vi "Double FFT Mesurament RT with Frequency Linearization.vi"() -> ()   [LabVIEW 2014]
uses:
  <vilib>/Platform/TimedLoop/XDataNode/timing_clust.ctl
  <vilib>/Platform/TimedLoop/XDataNode/nitl_modes.ctl
  <vilib>/Platform/TimedLoop/XDataNode/wakeup.ctl
  <vilib>/FPGAPlugInAG/sbRIO-9636/niLvFpga_Open_sbRIO-9636.vi
  <vilib>/rvi/interface/common/dynamic/niFpgaDynamicAddResources.vi
  <vilib>/Utility/error.llb/Error Cluster From Error Code.vi
  <vilib>/rvi/errors/niLvFpgaAdjustHostInterfaceError.vi
  <vilib>/rvi/interface/common/niFpgaWaitOnOcc.vi
  <vilib>/FPGAPlugInAG/Dynamic/niLvFpga_Run_Dynamic.vi
  <vilib>/FPGAPlugInAG/Dynamic/niLvFpga_Abort_Dynamic.vi
  <vilib>/FPGAPlugInAG/Dynamic/niLvFpga_Reset_Dynamic.vi
  <vilib>/FPGAPlugInAG/Dynamic/niLvFpga_Close_Dynamic.vi
  <vilib>/rvi/interface/nirviOpenFPGA/nirviOpenFPGA.xnode
  FPGA Bitfiles/LaserDistanceSen_FPGATarget_DoubleFFTMesuram_r82pz3ZO4sk.lvbitx
  FPGA Target/Test VIs/Double FFT Mesurament Test.vi
  FPGA Bitfiles/LaserDistanceSen_FPGATarget_DoubleFFTMesuram_atjrRfXVdPQ.lvbitx
  FPGA Target/Test VIs/Double FFT Mesurament Test SLOW.vi
  <vilib>/rvi/interface/nirviReadWriteControl/nirviReadWriteControl.xnode
  <vilib>/rvi/interface/nirviMethod/nirviMethod.xnode
  <vilib>/Platform/TimedLoop/XDataNode/XDataNode.xnode
  <vilib>/rvi/interface/nirviCloseFPGA/nirviCloseFPGA.xnode
  <vilib>/FPGAPlugInAG/Dynamic/niLvFpga_ConfigureFifo_Dynamic.vi
  <vilib>/rvi/errors/niLvFpgaMergeErrorWithErrorCode.vi
  <vilib>/FPGAPlugInAG/Dynamic/niLvFpga_StartFifo_Dynamic.vi
  <vilib>/rvi/interface/Simulation/niFpgaSimulationCallBeginRW.vi
  <vilib>/FPGAPlugInAG/Dynamic/niLvFpga_ReadFifo_Dynamic.vi
  <vilib>/Platform/TimedLoop/XDataNode/XDNodeRunTimeDep.lvlib
  NiFpgaLv.dll
panel:
  in  "Active PolyFit":bool
  out "2) Max-Min error":dbl
  out "1) Max-Min error":dbl
  in  "Sample /Modulation Frequency":enum32{"40MHz/32KHz", "30MHz/24Khz"}(radio)=enum."30MHz/24Khz"
  in  "Scaling Factor":dbl=1.0
  in  "Scale Factor Rising":dbl=0.5
  out "2) Std Dev":dbl
  out "1) Std Dev":dbl
  in  "Scale Factor Falling":dbl=0.5
  in  "Triangolo dritto":bool=TRUE
  in  "Acrive  Smooth":bool
  out "Complete SkewTri":dbl[](graph)
  out "2) Tri edge RISING":dbl[](graph)
  out "1) Tri edge FALLING":dbl[](graph)
  out "1) Ext Mean Time Curve":dbl[](graph)
  out "2) Ext Mean Time Curve":dbl[](graph)
  out "2) Mean Freq Curve Rising":dbl[](graph)
  out "1) Mean Freq Curve Falling":dbl[](graph)
  out "2) Freq curve":dbl[](graph)
  out "1) Freq curve":dbl[](graph)
  in  "FFT Sliding Win Size":i32=128
  out "1) SmoothSubSig":dbl[](graph)
  out "2) SmoothSubSig":dbl[](graph)
  in  "Acrive Fit":bool=TRUE
  in  "Poly Order":i32=3
  in  "Side points":i32=13
  in  "Poly Grade":dbl=5.0
  out "2) Signal&Fit 2":dbl[][](graph)
  out "1) Signal&Fit":dbl[][](graph)
  in  "tieni premuto per":i32=1
  out "Current Sig lin":i32
  in  "Acrive Linearization":bool
  in  "# Measurements for Linearization":i32=10
  in  "?":bool
  out "maxbin_secondFFT":i32
  out "maxbin_firstFFT":i32
  out "f_rise":dbl
  out "f_fall":dbl
  out "f_mean":dbl
  out "Velocity (m/s)":dbl
  out "Distance (m)":dbl
  in  "Initial Latency points":u32(slide) scale=0.0..1249.0
  out "Second FFT (bin)":dbl[](graph)
  out "Second Signal (points) - Rising Triangular":dbl[](graph)
  out "First FFT (bin)":dbl[](graph)
  out "First Signal (points) - Falling Triangular":dbl[](graph)
  in  "Snapshot":bool
  in  "Windowing":T1(ring)
  in  "first bin":i32=5
  in  "last bin":i32=255
  in  "lower limit 2":u32(slide)=738 scale=625.0..738.0
  in  "lower limit 1":u32(slide)=113 scale=0.0..113.0
  # "OFFLINE parameters"
  # "WARNING:\nOnce pressed wait untill the end of operation"
  # "Triangolo storto\nda costante"
  # "Max Detection FFT bin range"
  # "ONLINE parameters"
  # "Se la sottrazione del fondo non è eseguita su FPGA.\n Attivarla per eseguirla lato RT"
  # "Smoothing (S-G Params)"
  # "Fitting"
  # "ONLY POWER OF 2"
  # "Min: 2 Max: 256 (2, 4, 8, 16, 32, 64, 128, 256)"
  # "LINEARIZATION FINAL RESULTS"
  # "%"
  # "%"
  # "% over Mean"
  # "% over Mean"
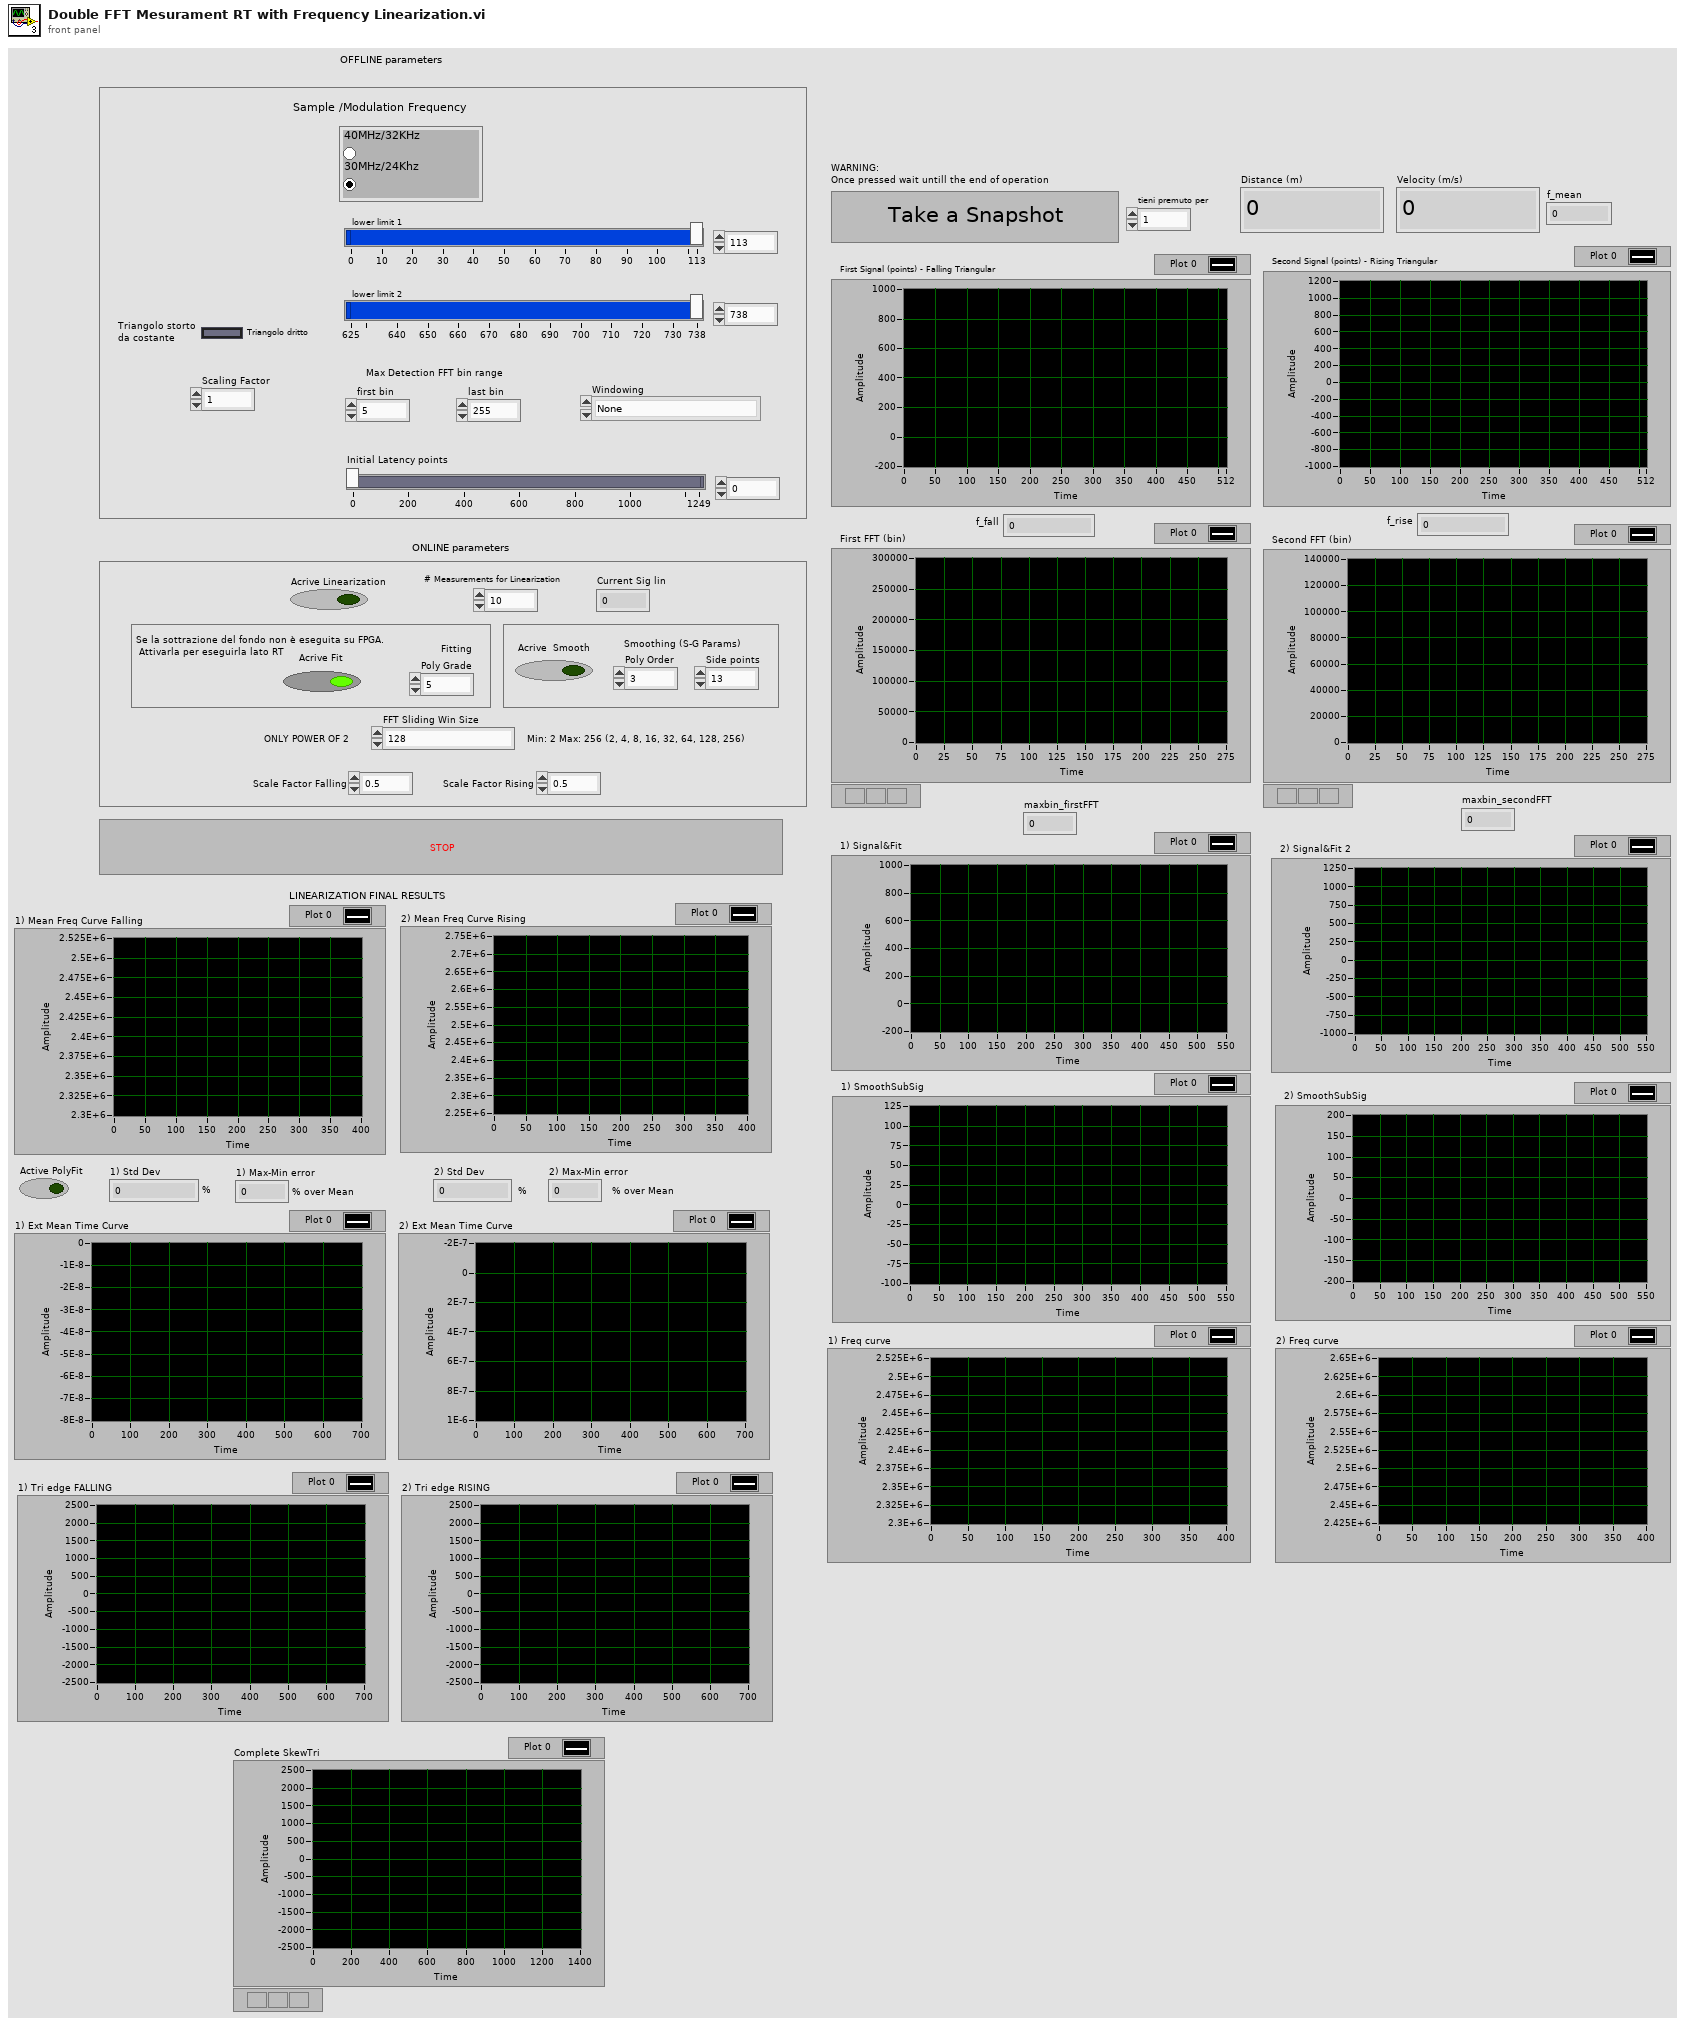
[diagram p1: front panel]
types:
  T1 = enum16{"None", "Hanning", "Hamming", "Blackman", "Blackman-Harris"}
  T2 = typedef "XDNodeRunTimeDep.lvlib/timing_clust.ctl" = cluster{"Expected End [f-1]":u64, "Actual End [f-1]":u64, "Finished Late? [f-1]":bool, "Expected End [i-1]":u64, "Actual End [i-1]":u64, "Finished Late? [i-1]":bool, "Expected Start [i]":u64, "Actual Start [i]":u64, "Expected Start [f]":u64, "Actual Start [f]":u64, "Source Name":string, "Structure Name":string, "Period":i64, "Deadline":i64, "Offset":i64, "Start":i64, "Priority":i32, "Timeout":i32, "Mode":T3, "Wakeup Reason":T4, "Error":errorcluster, "Source Type":string, "Secondary Source Type":string, "Global End Time":u64, "Global Start Time":u64, "Frame Duration":u64, "Iteration Duration":u64, "Assigned CPU":i32, "I/O Scan Engine Mode":u32}
  T3 = typedef "XDNodeRunTimeDep.lvlib/nitl_modes.ctl" = enum32{"No Change", "Process missed periods, maintain original phase", "Discard missed periods, maintain original phase", "Process missed periods, ignore original phase", "Discard missed periods, ignore original phase"}
  T4 = typedef "XDNodeRunTimeDep.lvlib/wakeup.ctl" = enum32{"Normal", "Aborted", "Asynchronous wakeup", "Timing source error", "Timed loop error", "Timeout"}
  T5 = typedef "NI_Matrix.lvlib/RealMatrix.ctl" = dbl[][]
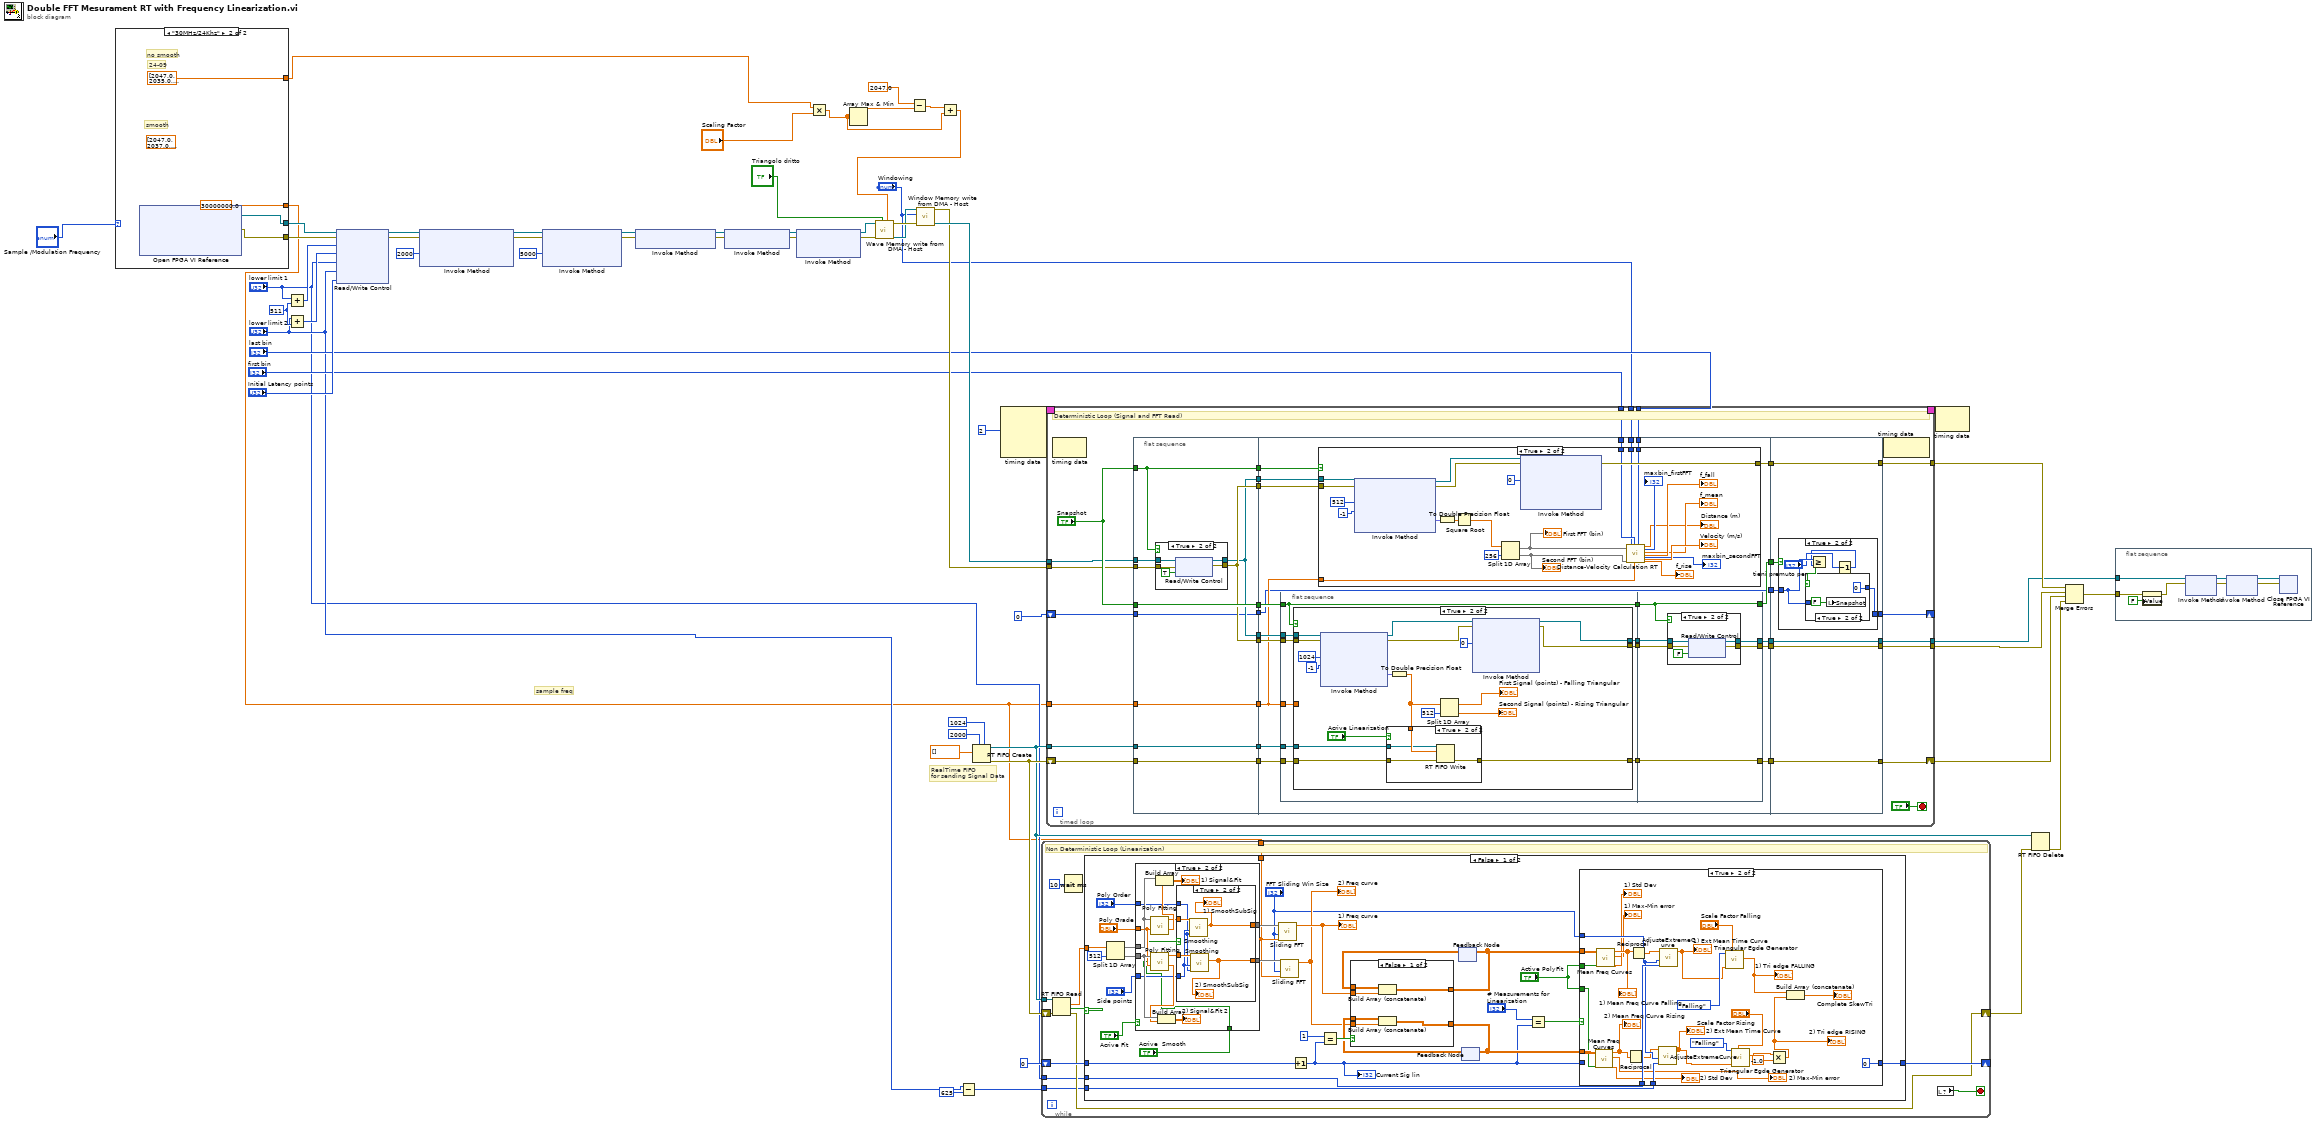
[diagram p0: block diagram]
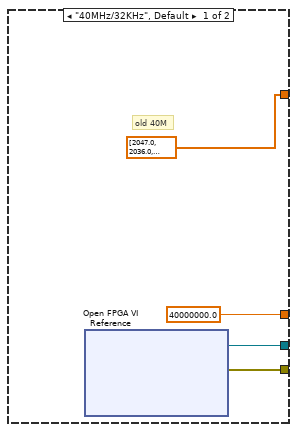
[diagram p2: hidden frame]
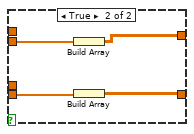
[diagram p6: hidden frame]
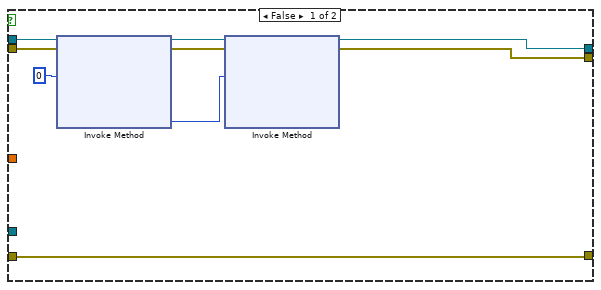
[diagram p9: hidden frame]
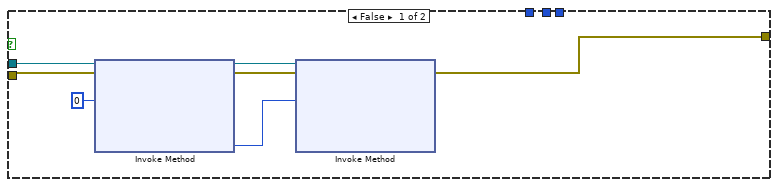
[diagram p12: hidden frame]
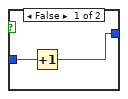
[diagram p14: hidden frame]
diagram:
  w56 = u32 511 ("y")
  # "sample freq"
  # "RealTime FIFO \nfor sending Signal Data"
  n1 = case shown="\"30MHz/24Khz\"" "Sample /Modulation Frequency" {
    tunnel: [w62 w65] -> w55
    tunnel: [w61 w66] -> w54
    tunnel: [40000000.0 30000000.0] -> w2
    tunnel: [dbl[] [2047.0, 2036.0, 2024.0, 2013.0, 2002.0, 1990.0, 1979.0, 1968.0, 1956.0, 1945.0, 1934.0, 1923.0, 1912.0, 1900.0, 1889.0, 1878.0, 1867.0, 1856.0, 1845.0, 1833.0, 1822.0, 1811.0, 1800.0, 1789.0, 1778.0, 1767.0, 1756.0, 1745.0, 1734.0, 1723.0, 1712.0, 1702.0, 1691.0, 1680.0, 1669.0, 1658.0, 1647.0, 1636.0, 1626.0, 1615.0, 1604.0, 1593.0, 1583.0, 1572.0, 1561.0, 1550.0, 1540.0, 1529.0, 1518.0, 1508.0, 1497.0, 1487.0, 1476.0, 1465.0, 1455.0, 1444.0, 1434.0, 1423.0, 1413.0, 1402.0, 1392.0, 1381.0, 1371.0, 1360.0, 1350.0, 1340.0, 1329.0, 1319.0, 1309.0, 1298.0, 1288.0, 1278.0, 1267.0, 1257.0, 1247.0, 1237.0, 1226.0, 1216.0, 1206.0, 1196.0, 1186.0, 1176.0, 1165.0, 1155.0, 1145.0, 1135.0, 1125.0, 1115.0, 1105.0, 1095.0, 1085.0, 1075.0, 1065.0, 1055.0, 1045.0, 1035.0, 1025.0, 1015.0, 1006.0, 996.0, 986.0, 976.0, 966.0, 956.0, 947.0, 937.0, 927.0, 917.0, 908.0, 898.0, 888.0, 879.0, 869.0, 859.0, 850.0, 837.0, 826.0, 816.0, 804.0, 796.0, 788.0, 778.0, 769.0, 758.0, 750.0, 743.0, 733.0, 724.0, 717.0, 709.0, 701.0, 693.0, 686.0, 677.0, 669.0, 661.0, 653.0, 645.0, 638.0, 630.0, 622.0, 615.0, 607.0, 599.0, 592.0, 583.0, 576.0, 569.0, 561.0, 554.0, 547.0, 539.0, 532.0, 525.0, 518.0, 509.0, 501.0, 492.0, 486.0, 478.0, 471.0, 463.0, 456.0, 450.0, 442.0, 435.0, 429.0, 421.0, 415.0, 408.0, 401.0, 394.0, 388.0, 381.0, 375.0, 368.0, 361.0, 355.0, 349.0, 342.0, 336.0, 330.0, 323.0, 317.0, 311.0, 304.0, 298.0, 292.0, 286.0, 279.0, 273.0, 267.0, 261.0, 255.0, 249.0, 242.0, 236.0, 230.0, 224.0, 218.0, 212.0, 206.0, 200.0, 194.0, 187.0, 181.0, 175.0, 169.0, 163.0, 157.0, 150.0, 144.0, 138.0, 132.0, 125.0, 119.0, 113.0, 107.0, 101.0, 95.0, 88.0, 82.0, 77.0, 71.0, 65.0, 59.0, 53.0, 47.0, 41.0, 35.0, 29.0, 23.0, 18.0, 11.0, 6.0, 0.0, -6.0, -12.0, -18.0, -23.0, -29.0, -35.0, -41.0, -47.0, -52.0, -58.0, -64.0, -69.0, -75.0, -81.0, -87.0, -92.0, -98.0, -104.0, -109.0, -115.0, -121.0, -126.0, -132.0, -138.0, -144.0, -149.0, -155.0, -161.0, -166.0, -172.0, -177.0, -183.0, -189.0, -194.0, -200.0, -205.0, -211.0, -216.0, -222.0, -227.0, -233.0, -238.0, -244.0, -249.0, -255.0, -260.0, -266.0, -271.0, -277.0, -283.0, -288.0, -294.0, -299.0, -304.0, -310.0, -315.0, -321.0, -326.0, -331.0, -337.0, -342.0, -348.0, -353.0, -358.0, -364.0, -369.0, -375.0, -380.0, -385.0, -391.0, -396.0, -402.0, -407.0, -413.0, -418.0, -423.0, -429.0, -434.0, -439.0, -445.0, -450.0, -456.0, -461.0, -466.0, -472.0, -477.0, -483.0, -488.0, -493.0, -499.0, -504.0, -510.0, -515.0, -520.0, -526.0, -531.0, -537.0, -542.0, -548.0, -553.0, -558.0, -564.0, -569.0, -574.0, -580.0, -585.0, -590.0, -596.0, -601.0, -606.0, -612.0, -617.0, -622.0, -628.0, -633.0, -638.0, -644.0, -649.0, -654.0, -660.0, -665.0, -670.0, -676.0, -681.0, -686.0, -692.0, -697.0, -702.0, -708.0, -713.0, -718.0, -723.0, -729.0, -734.0, -739.0, -744.0, -750.0, -755.0, -760.0, -765.0, -771.0, -776.0, -781.0, -786.0, -792.0, -797.0, -802.0, -807.0, -812.0, -818.0, -823.0, -828.0, -833.0, -839.0, -844.0, -849.0, -854.0, -859.0, -865.0, -870.0, -875.0, -880.0, -885.0, -891.0, -896.0, -901.0, -906.0, -911.0, -916.0, -922.0, -927.0, -932.0, -937.0, -943.0, -948.0, -953.0, -958.0, -963.0, -969.0, -974.0, -979.0, -984.0, -989.0, -995.0, -1000.0, -1005.0, -1010.0, -1015.0, -1021.0, -1026.0, -1031.0, -1036.0, -1041.0, -1047.0, -1052.0, -1057.0, -1062.0, -1067.0, -1073.0, -1078.0, -1083.0, -1088.0, -1093.0, -1099.0, -1104.0, -1109.0, -1114.0, -1119.0, -1124.0, -1130.0, -1135.0, -1140.0, -1145.0, -1150.0, -1156.0, -1161.0, -1166.0, -1171.0, -1176.0, -1182.0, -1187.0, -1192.0, -1197.0, -1202.0, -1207.0, -1213.0, -1218.0, -1223.0, -1228.0, -1233.0, -1238.0, -1244.0, -1249.0, -1254.0, -1259.0, -1264.0, -1269.0, -1275.0, -1280.0, -1285.0, -1290.0, -1295.0, -1300.0, -1305.0, -1311.0, -1316.0, -1321.0, -1326.0, -1331.0, -1336.0, -1342.0, -1347.0, -1352.0, -1357.0, -1362.0, -1367.0, -1372.0, -1378.0, -1383.0, -1388.0, -1393.0, -1398.0, -1403.0, -1408.0, -1414.0, -1419.0, -1424.0, -1429.0, -1434.0, -1439.0, -1444.0, -1450.0, -1455.0, -1460.0, -1465.0, -1470.0, -1475.0, -1480.0, -1486.0, -1491.0, -1496.0, -1501.0, -1506.0, -1511.0, -1516.0, -1522.0, -1527.0, -1532.0, -1537.0, -1542.0, -1547.0, -1552.0, -1558.0, -1563.0, -1568.0, -1573.0, -1578.0, -1583.0, -1588.0, -1593.0, -1599.0, -1604.0, -1609.0, -1614.0, -1619.0, -1624.0, -1629.0, -1634.0, -1640.0, -1645.0, -1650.0, -1655.0, -1660.0, -1665.0, -1670.0, -1675.0, -1681.0, -1686.0, -1691.0, -1696.0, -1701.0, -1706.0, -1711.0, -1716.0, -1722.0, -1727.0, -1732.0, -1737.0, -1742.0, -1747.0, -1752.0, -1757.0, -1762.0, -1768.0, -1773.0, -1778.0, -1783.0, -1788.0, -1793.0, -1798.0, -1803.0, -1808.0, -1814.0, -1819.0, -1824.0, -1829.0, -1834.0, -1839.0, -1844.0, -1849.0, -1854.0, -1859.0, -1865.0, -1870.0, -1875.0, -1880.0, -1885.0, -1890.0, -1895.0, -1900.0, -1905.0, -1911.0, -1916.0, -1921.0, -1926.0, -1931.0, -1936.0, -1941.0, -1946.0, -1951.0, -1956.0, -1961.0, -1967.0, -1972.0, -1977.0, -1982.0, -1987.0, -1992.0, -1997.0, -2002.0, -2007.0, -2012.0, -2017.0, -2023.0, -2028.0, -2033.0, -2038.0, -2043.0, -2048.0, -2047.0, -2034.0, -2021.0, -2009.0, -1996.0, -1983.0, -1970.0, -1957.0, -1945.0, -1932.0, -1919.0, -1907.0, -1894.0, -1881.0, -1869.0, -1856.0, -1844.0, -1831.0, -1819.0, -1806.0, -1794.0, -1781.0, -1769.0, -1757.0, -1744.0, -1732.0, -1719.0, -1707.0, -1695.0, -1682.0, -1670.0, -1658.0, -1646.0, -1634.0, -1621.0, -1609.0, -1597.0, -1585.0, -1573.0, -1561.0, -1549.0, -1537.0, -1525.0, -1513.0, -1501.0, -1489.0, -1477.0, -1465.0, -1453.0, -1441.0, -1429.0, -1417.0, -1405.0, -1394.0, -1382.0, -1370.0, -1358.0, -1347.0, -1335.0, -1323.0, -1312.0, -1300.0, -1288.0, -1277.0, -1265.0, -1254.0, -1242.0, -1231.0, -1219.0, -1208.0, -1196.0, -1185.0, -1173.0, -1162.0, -1150.0, -1139.0, -1128.0, -1116.0, -1105.0, -1094.0, -1083.0, -1071.0, -1060.0, -1049.0, -1038.0, -1027.0, -1015.0, -1004.0, -993.0, -982.0, -971.0, -960.0, -949.0, -938.0, -927.0, -916.0, -905.0, -894.0, -883.0, -873.0, -862.0, -851.0, -840.0, -829.0, -819.0, -808.0, -797.0, -786.0, -776.0, -765.0, -754.0, -744.0, -733.0, -722.0, -712.0, -697.0, -685.0, -674.0, -661.0, -652.0, -643.0, -632.0, -622.0, -610.0, -602.0, -594.0, -583.0, -574.0, -566.0, -558.0, -550.0, -542.0, -534.0, -525.0, -516.0, -507.0, -499.0, -491.0, -483.0, -475.0, -467.0, -459.0, -451.0, -443.0, -435.0, -426.0, -419.0, -411.0, -404.0, -396.0, -388.0, -381.0, -373.0, -366.0, -359.0, -349.0, -341.0, -331.0, -325.0, -317.0, -309.0, -301.0, -295.0, -288.0, -280.0, -273.0, -266.0, -259.0, -252.0, -246.0, -239.0, -231.0, -225.0, -219.0, -212.0, -205.0, -199.0, -192.0, -186.0, -180.0, -173.0, -167.0, -161.0, -155.0, -148.0, -142.0, -136.0, -130.0, -124.0, -118.0, -112.0, -106.0, -100.0, -94.0, -88.0, -82.0, -76.0, -70.0, -64.0, -58.0, -52.0, -46.0, -40.0, -34.0, -28.0, -21.0, -15.0, -9.0, -3.0, 2.0, 9.0, 15.0, 21.0, 27.0, 33.0, 39.0, 45.0, 51.0, 57.0, 63.0, 69.0, 75.0, 81.0, 86.0, 92.0, 98.0, 103.0, 110.0, 116.0, 121.0, 127.0, 133.0, 138.0, 144.0, 149.0, 155.0, 161.0, 166.0, 172.0, 177.0, 183.0, 189.0, 194.0, 200.0, 205.0, 211.0, 216.0, 221.0, 227.0, 232.0, 238.0, 243.0, 249.0, 254.0, 259.0, 265.0, 270.0, 276.0, 281.0, 286.0, 292.0, 297.0, 303.0, 308.0, 314.0, 319.0, 324.0, 329.0, 335.0, 340.0, 345.0, 351.0, 356.0, 361.0, 366.0, 371.0, 377.0, 382.0, 387.0, 392.0, 397.0, 403.0, 408.0, 413.0, 418.0, 423.0, 429.0, 434.0, 439.0, 444.0, 449.0, 454.0, 459.0, 464.0, 469.0, 474.0, 479.0, 484.0, 489.0, 494.0, 499.0, 504.0, 509.0, 514.0, 520.0, 525.0, 530.0, 535.0, 540.0, 545.0, 550.0, 555.0, 560.0, 565.0, 570.0, 575.0, 580.0, 585.0, 590.0, 595.0, 600.0, 605.0, 610.0, 615.0, 620.0, 625.0, 630.0, 636.0, 641.0, 646.0, 651.0, 656.0, 661.0, 666.0, 671.0, 676.0, 681.0, 686.0, 691.0, 696.0, 701.0, 706.0, 711.0, 716.0, 721.0, 726.0, 731.0, 736.0, 741.0, 746.0, 751.0, 756.0, 761.0, 765.0, 770.0, 775.0, 780.0, 785.0, 790.0, 795.0, 800.0, 805.0, 810.0, 815.0, 820.0, 825.0, 829.0, 834.0, 839.0, 844.0, 849.0, 854.0, 859.0, 864.0, 868.0, 873.0, 878.0, 883.0, 888.0, 893.0, 897.0, 902.0, 907.0, 912.0, 917.0, 921.0, 926.0, 931.0, 936.0, 941.0, 945.0, 950.0, 955.0, 960.0, 965.0, 969.0, 974.0, 979.0, 984.0, 988.0, 993.0, 998.0, 1003.0, 1007.0, 1012.0, 1017.0, 1022.0, 1027.0, 1031.0, 1036.0, 1041.0, 1046.0, 1051.0, 1055.0, 1060.0, 1065.0, 1070.0, 1075.0, 1079.0, 1084.0, 1089.0, 1094.0, 1098.0, 1103.0, 1108.0, 1113.0, 1118.0, 1122.0, 1127.0, 1132.0, 1137.0, 1141.0, 1146.0, 1151.0, 1156.0, 1161.0, 1165.0, 1170.0, 1175.0, 1180.0, 1184.0, 1189.0, 1194.0, 1199.0, 1204.0, 1208.0, 1213.0, 1218.0, 1223.0, 1227.0, 1232.0, 1237.0, 1242.0, 1246.0, 1251.0, 1256.0, 1261.0, 1265.0, 1270.0, 1275.0, 1280.0, 1284.0, 1289.0, 1294.0, 1299.0, 1303.0, 1308.0, 1313.0, 1318.0, 1322.0, 1327.0, 1332.0, 1336.0, 1341.0, 1346.0, 1351.0, 1355.0, 1360.0, 1365.0, 1370.0, 1374.0, 1379.0, 1384.0, 1388.0, 1393.0, 1398.0, 1403.0, 1407.0, 1412.0, 1417.0, 1421.0, 1426.0, 1431.0, 1436.0, 1440.0, 1445.0, 1450.0, 1454.0, 1459.0, 1464.0, 1469.0, 1473.0, 1478.0, 1483.0, 1487.0, 1492.0, 1497.0, 1502.0, 1506.0, 1511.0, 1516.0, 1520.0, 1525.0, 1530.0, 1535.0, 1539.0, 1544.0, 1549.0, 1553.0, 1558.0, 1563.0, 1567.0, 1572.0, 1577.0, 1582.0, 1586.0, 1591.0, 1596.0, 1600.0, 1605.0, 1610.0, 1614.0, 1619.0, 1624.0, 1628.0, 1633.0, 1638.0, 1643.0, 1647.0, 1652.0, 1657.0, 1661.0, 1666.0, 1671.0, 1675.0, 1680.0, 1685.0, 1689.0, 1694.0, 1699.0, 1703.0, 1708.0, 1713.0, 1717.0, 1722.0, 1727.0, 1731.0, 1736.0, 1741.0, 1746.0, 1750.0, 1755.0, 1760.0, 1764.0, 1769.0, 1774.0, 1778.0, 1783.0, 1788.0, 1792.0, 1797.0, 1802.0, 1806.0, 1811.0, 1816.0, 1820.0, 1825.0, 1830.0, 1834.0, 1839.0, 1844.0, 1848.0, 1853.0, 1858.0, 1862.0, 1867.0, 1871.0, 1876.0, 1881.0, 1885.0, 1890.0, 1895.0, 1899.0, 1904.0, 1909.0, 1913.0, 1918.0, 1923.0, 1927.0, 1932.0, 1937.0, 1941.0, 1946.0, 1951.0, 1955.0, 1960.0, 1965.0, 1969.0, 1974.0, 1978.0, 1983.0, 1988.0, 1992.0, 1997.0, 2002.0, 2006.0, 2011.0, 2016.0, 2020.0, 2025.0, 2029.0, 2034.0, 2039.0, 2043.0, 2048.0] ("Complete SkewTri") dbl[] [2047.0, 2035.0, 2022.0, 2010.0, 1997.0, 1985.0, 1972.0, 1960.0, 1948.0, 1935.0, 1923.0, 1911.0, 1899.0, 1886.0, 1874.0, 1862.0, 1850.0, 1838.0, 1825.0, 1813.0, 1801.0, 1789.0, 1777.0, 1765.0, 1753.0, 1741.0, 1729.0, 1717.0, 1705.0, 1693.0, 1681.0, 1669.0, 1657.0, 1645.0, 1634.0, 1622.0, 1610.0, 1598.0, 1586.0, 1575.0, 1563.0, 1551.0, 1540.0, 1528.0, 1516.0, 1505.0, 1493.0, 1481.0, 1470.0, 1458.0, 1447.0, 1435.0, 1424.0, 1412.0, 1401.0, 1389.0, 1378.0, 1366.0, 1355.0, 1344.0, 1332.0, 1321.0, 1310.0, 1298.0, 1287.0, 1276.0, 1265.0, 1253.0, 1242.0, 1231.0, 1220.0, 1209.0, 1198.0, 1186.0, 1175.0, 1164.0, 1153.0, 1142.0, 1131.0, 1120.0, 1109.0, 1098.0, 1087.0, 1076.0, 1065.0, 1055.0, 1044.0, 1033.0, 1022.0, 1011.0, 1000.0, 990.0, 979.0, 968.0, 958.0, 947.0, 936.0, 926.0, 915.0, 904.0, 894.0, 883.0, 873.0, 862.0, 852.0, 841.0, 831.0, 820.0, 810.0, 799.0, 789.0, 778.0, 768.0, 758.0, 747.0, 738.0, 727.0, 719.0, 712.0, 706.0, 700.0, 693.0, 687.0, 680.0, 674.0, 668.0, 661.0, 655.0, 648.0, 642.0, 636.0, 629.0, 623.0, 617.0, 610.0, 604.0, 598.0, 591.0, 584.0, 577.0, 569.0, 560.0, 552.0, 545.0, 538.0, 531.0, 525.0, 519.0, 512.0, 506.0, 500.0, 494.0, 488.0, 482.0, 476.0, 470.0, 464.0, 458.0, 452.0, 446.0, 436.0, 430.0, 424.0, 418.0, 412.0, 406.0, 400.0, 394.0, 388.0, 382.0, 376.0, 370.0, 364.0, 358.0, 352.0, 346.0, 338.0, 332.0, 325.0, 319.0, 313.0, 307.0, 301.0, 295.0, 290.0, 284.0, 278.0, 272.0, 267.0, 261.0, 255.0, 249.0, 244.0, 238.0, 232.0, 227.0, 221.0, 215.0, 209.0, 204.0, 198.0, 192.0, 187.0, 181.0, 175.0, 170.0, 164.0, 158.0, 153.0, 147.0, 141.0, 136.0, 130.0, 124.0, 119.0, 113.0, 108.0, 102.0, 96.0, 91.0, 85.0, 79.0, 74.0, 68.0, 62.0, 57.0, 51.0, 45.0, 39.0, 34.0, 28.0, 22.0, 16.0, 11.0, 5.0, 0.0, -6.0, -11.0, -17.0, -22.0, -28.0, -33.0, -39.0, -44.0, -50.0, -55.0, -61.0, -66.0, -72.0, -77.0, -83.0, -88.0, -94.0, -99.0, -105.0, -110.0, -116.0, -121.0, -127.0, -132.0, -137.0, -143.0, -148.0, -154.0, -159.0, -165.0, -170.0, -176.0, -181.0, -186.0, -192.0, -197.0, -203.0, -208.0, -214.0, -219.0, -224.0, -230.0, -235.0, -241.0, -246.0, -251.0, -257.0, -262.0, -268.0, -273.0, -278.0, -284.0, -289.0, -295.0, -300.0, -305.0, -311.0, -316.0, -321.0, -327.0, -332.0, -337.0, -343.0, -348.0, -354.0, -359.0, -364.0, -370.0, -375.0, -380.0, -386.0, -391.0, -397.0, -402.0, -407.0, -413.0, -418.0, -423.0, -429.0, -434.0, -439.0, -445.0, -450.0, -455.0, -461.0, -466.0, -471.0, -477.0, -482.0, -487.0, -493.0, -498.0, -503.0, -509.0, -514.0, -519.0, -525.0, -530.0, -535.0, -540.0, -546.0, -551.0, -556.0, -562.0, -567.0, -572.0, -578.0, -583.0, -588.0, -593.0, -599.0, -604.0, -609.0, -615.0, -620.0, -625.0, -630.0, -636.0, -641.0, -646.0, -651.0, -657.0, -662.0, -667.0, -673.0, -678.0, -683.0, -688.0, -694.0, -699.0, -704.0, -709.0, -715.0, -720.0, -725.0, -730.0, -736.0, -741.0, -746.0, -751.0, -757.0, -762.0, -767.0, -772.0, -778.0, -783.0, -788.0, -793.0, -799.0, -804.0, -809.0, -814.0, -820.0, -825.0, -830.0, -835.0, -841.0, -846.0, -851.0, -856.0, -862.0, -867.0, -872.0, -877.0, -883.0, -888.0, -893.0, -898.0, -903.0, -909.0, -914.0, -919.0, -924.0, -930.0, -935.0, -940.0, -945.0, -951.0, -956.0, -961.0, -966.0, -971.0, -977.0, -982.0, -987.0, -992.0, -998.0, -1003.0, -1008.0, -1013.0, -1018.0, -1024.0, -1029.0, -1034.0, -1039.0, -1045.0, -1050.0, -1055.0, -1060.0, -1065.0, -1071.0, -1076.0, -1081.0, -1086.0, -1092.0, -1097.0, -1102.0, -1107.0, -1112.0, -1118.0, -1123.0, -1128.0, -1133.0, -1138.0, -1144.0, -1149.0, -1154.0, -1159.0, -1165.0, -1170.0, -1175.0, -1180.0, -1185.0, -1191.0, -1196.0, -1201.0, -1206.0, -1211.0, -1217.0, -1222.0, -1227.0, -1232.0, -1237.0, -1243.0, -1248.0, -1253.0, -1258.0, -1263.0, -1269.0, -1274.0, -1279.0, -1284.0, -1289.0, -1295.0, -1300.0, -1305.0, -1310.0, -1315.0, -1321.0, -1326.0, -1331.0, -1336.0, -1341.0, -1347.0, -1352.0, -1357.0, -1362.0, -1367.0, -1373.0, -1378.0, -1383.0, -1388.0, -1393.0, -1399.0, -1404.0, -1409.0, -1414.0, -1419.0, -1425.0, -1430.0, -1435.0, -1440.0, -1445.0, -1450.0, -1456.0, -1461.0, -1466.0, -1471.0, -1476.0, -1482.0, -1487.0, -1492.0, -1497.0, -1502.0, -1508.0, -1513.0, -1518.0, -1523.0, -1528.0, -1534.0, -1539.0, -1544.0, -1549.0, -1554.0, -1560.0, -1565.0, -1570.0, -1575.0, -1580.0, -1586.0, -1591.0, -1596.0, -1601.0, -1606.0, -1612.0, -1617.0, -1622.0, -1627.0, -1632.0, -1637.0, -1643.0, -1648.0, -1653.0, -1658.0, -1663.0, -1669.0, -1674.0, -1679.0, -1684.0, -1689.0, -1695.0, -1700.0, -1705.0, -1710.0, -1715.0, -1721.0, -1726.0, -1731.0, -1736.0, -1741.0, -1747.0, -1752.0, -1757.0, -1762.0, -1767.0, -1773.0, -1778.0, -1783.0, -1788.0, -1793.0, -1799.0, -1804.0, -1809.0, -1814.0, -1819.0, -1825.0, -1830.0, -1835.0, -1840.0, -1845.0, -1851.0, -1856.0, -1861.0, -1866.0, -1871.0, -1876.0, -1882.0, -1887.0, -1892.0, -1897.0, -1902.0, -1908.0, -1913.0, -1918.0, -1923.0, -1928.0, -1934.0, -1939.0, -1944.0, -1949.0, -1954.0, -1960.0, -1965.0, -1970.0, -1975.0, -1980.0, -1986.0, -1991.0, -1996.0, -2001.0, -2006.0, -2012.0, -2017.0, -2022.0, -2027.0, -2032.0, -2038.0, -2043.0, -2048.0, -2047.0, -2037.0, -2027.0, -2017.0, -2007.0, -1997.0, -1987.0, -1977.0, -1967.0, -1957.0, -1947.0, -1937.0, -1927.0, -1917.0, -1907.0, -1897.0, -1888.0, -1878.0, -1868.0, -1858.0, -1848.0, -1838.0, -1828.0, -1819.0, -1809.0, -1799.0, -1789.0, -1780.0, -1770.0, -1760.0, -1750.0, -1741.0, -1731.0, -1721.0, -1712.0, -1702.0, -1692.0, -1683.0, -1673.0, -1663.0, -1654.0, -1644.0, -1635.0, -1625.0, -1615.0, -1606.0, -1596.0, -1587.0, -1577.0, -1568.0, -1558.0, -1549.0, -1539.0, -1530.0, -1520.0, -1511.0, -1501.0, -1492.0, -1483.0, -1473.0, -1464.0, -1454.0, -1445.0, -1436.0, -1426.0, -1417.0, -1408.0, -1398.0, -1389.0, -1380.0, -1371.0, -1361.0, -1352.0, -1343.0, -1334.0, -1324.0, -1315.0, -1306.0, -1297.0, -1288.0, -1278.0, -1269.0, -1260.0, -1251.0, -1242.0, -1233.0, -1224.0, -1215.0, -1205.0, -1196.0, -1187.0, -1178.0, -1169.0, -1160.0, -1151.0, -1142.0, -1133.0, -1124.0, -1115.0, -1106.0, -1097.0, -1088.0, -1080.0, -1071.0, -1062.0, -1053.0, -1044.0, -1035.0, -1026.0, -1017.0, -1009.0, -1000.0, -991.0, -982.0, -973.0, -965.0, -953.0, -944.0, -935.0, -920.0, -906.0, -889.0, -871.0, -854.0, -842.0, -834.0, -826.0, -818.0, -810.0, -802.0, -794.0, -786.0, -778.0, -770.0, -762.0, -754.0, -746.0, -739.0, -731.0, -723.0, -715.0, -707.0, -699.0, -690.0, -682.0, -672.0, -661.0, -651.0, -639.0, -627.0, -616.0, -606.0, -598.0, -591.0, -584.0, -577.0, -570.0, -563.0, -556.0, -549.0, -542.0, -535.0, -528.0, -520.0, -513.0, -506.0, -499.0, -492.0, -485.0, -478.0, -471.0, -464.0, -457.0, -451.0, -444.0, -437.0, -430.0, -423.0, -416.0, -409.0, -400.0, -390.0, -382.0, -373.0, -364.0, -356.0, -349.0, -343.0, -336.0, -330.0, -323.0, -317.0, -310.0, -304.0, -297.0, -291.0, -284.0, -278.0, -271.0, -265.0, -258.0, -252.0, -245.0, -239.0, -232.0, -226.0, -219.0, -213.0, -207.0, -200.0, -194.0, -187.0, -181.0, -175.0, -168.0, -162.0, -156.0, -149.0, -143.0, -136.0, -128.0, -121.0, -114.0, -107.0, -100.0, -93.0, -87.0, -80.0, -74.0, -68.0, -62.0, -56.0, -50.0, -44.0, -38.0, -32.0, -26.0, -20.0, -14.0, -8.0, -2.0, 5.0, 11.0, 17.0, 23.0, 29.0, 35.0, 41.0, 47.0, 53.0, 59.0, 65.0, 70.0, 76.0, 82.0, 88.0, 94.0, 100.0, 106.0, 112.0, 118.0, 124.0, 130.0, 136.0, 142.0, 148.0, 154.0, 161.0, 167.0, 174.0, 180.0, 186.0, 192.0, 198.0, 204.0, 210.0, 215.0, 221.0, 227.0, 233.0, 238.0, 244.0, 250.0, 255.0, 261.0, 267.0, 273.0, 278.0, 284.0, 290.0, 295.0, 301.0, 307.0, 312.0, 318.0, 324.0, 329.0, 335.0, 341.0, 346.0, 352.0, 358.0, 363.0, 369.0, 374.0, 380.0, 386.0, 391.0, 397.0, 402.0, 408.0, 414.0, 419.0, 425.0, 430.0, 436.0, 441.0, 447.0, 453.0, 458.0, 464.0, 470.0, 475.0, 481.0, 487.0, 493.0, 499.0, 504.0, 510.0, 516.0, 521.0, 527.0, 532.0, 538.0, 543.0, 549.0, 554.0, 560.0, 565.0, 571.0, 576.0, 582.0, 587.0, 593.0, 598.0, 604.0, 609.0, 614.0, 620.0, 625.0, 631.0, 636.0, 642.0, 647.0, 653.0, 658.0, 663.0, 669.0, 674.0, 680.0, 685.0, 691.0, 696.0, 701.0, 707.0, 712.0, 718.0, 723.0, 728.0, 734.0, 739.0, 745.0, 750.0, 755.0, 761.0, 766.0, 772.0, 777.0, 782.0, 788.0, 793.0, 798.0, 804.0, 809.0, 815.0, 820.0, 826.0, 831.0, 837.0, 842.0, 847.0, 853.0, 858.0, 863.0, 869.0, 874.0, 880.0, 885.0, 890.0, 895.0, 901.0, 906.0, 911.0, 917.0, 922.0, 927.0, 933.0, 938.0, 943.0, 948.0, 954.0, 959.0, 964.0, 970.0, 975.0, 980.0, 985.0, 991.0, 996.0, 1001.0, 1006.0, 1012.0, 1017.0, 1022.0, 1027.0, 1033.0, 1038.0, 1043.0, 1048.0, 1054.0, 1059.0, 1064.0, 1069.0, 1075.0, 1080.0, 1085.0, 1090.0, 1096.0, 1101.0, 1106.0, 1111.0, 1116.0, 1122.0, 1127.0, 1132.0, 1137.0, 1143.0, 1148.0, 1153.0, 1158.0, 1163.0, 1169.0, 1174.0, 1179.0, 1184.0, 1190.0, 1195.0, 1200.0, 1205.0, 1211.0, 1216.0, 1221.0, 1226.0, 1231.0, 1237.0, 1242.0, 1247.0, 1252.0, 1257.0, 1262.0, 1268.0, 1273.0, 1278.0, 1283.0, 1288.0, 1293.0, 1298.0, 1304.0, 1309.0, 1314.0, 1319.0, 1324.0, 1329.0, 1334.0, 1340.0, 1345.0, 1350.0, 1355.0, 1360.0, 1365.0, 1370.0, 1375.0, 1381.0, 1386.0, 1391.0, 1396.0, 1401.0, 1406.0, 1411.0, 1416.0, 1421.0, 1427.0, 1432.0, 1437.0, 1442.0, 1447.0, 1452.0, 1457.0, 1462.0, 1467.0, 1472.0, 1478.0, 1483.0, 1488.0, 1493.0, 1498.0, 1503.0, 1508.0, 1513.0, 1518.0, 1523.0, 1528.0, 1534.0, 1539.0, 1544.0, 1549.0, 1554.0, 1559.0, 1564.0, 1569.0, 1574.0, 1579.0, 1584.0, 1589.0, 1595.0, 1600.0, 1605.0, 1610.0, 1615.0, 1620.0, 1625.0, 1630.0, 1635.0, 1640.0, 1645.0, 1650.0, 1655.0, 1660.0, 1666.0, 1671.0, 1676.0, 1681.0, 1686.0, 1691.0, 1696.0, 1701.0, 1706.0, 1711.0, 1716.0, 1721.0, 1726.0, 1731.0, 1736.0, 1741.0, 1746.0, 1751.0, 1757.0, 1762.0, 1767.0, 1772.0, 1777.0, 1782.0, 1787.0, 1792.0, 1797.0, 1802.0, 1807.0, 1812.0, 1817.0, 1822.0, 1827.0, 1832.0, 1837.0, 1842.0, 1847.0, 1852.0, 1857.0, 1862.0, 1867.0, 1872.0, 1877.0, 1883.0, 1888.0, 1893.0, 1898.0, 1903.0, 1908.0, 1913.0, 1918.0, 1923.0, 1928.0, 1933.0, 1938.0, 1943.0, 1948.0, 1953.0, 1958.0, 1963.0, 1968.0, 1973.0, 1978.0, 1983.0, 1988.0, 1993.0, 1998.0, 2003.0, 2008.0, 2013.0, 2018.0, 2023.0, 2028.0, 2033.0, 2038.0, 2043.0, 2048.0] ("appended array")] -> w1
    frame "40MHz/32KHz", Default {
      # "old 40M"
      n2 = xnode "Open FPGA VI Reference"() -> ("FPGA VI Reference Out"=w62:refnum<k20>, "error out"=w61:errorcluster)  [unwired: 2 in]
    }
    frame "30MHz/24Khz" {
      (unwired) dbl[] [2047.0, 2037.0, 2027.0, 2018.0, 2008.0, 1998.0, 1989.0, 1979.0, 1969.0, 1960.0, 1950.0, 1940.0, 1931.0, 1921.0, 1911.0, 1902.0, 1892.0, 1882.0, 1873.0, 1863.0, 1854.0, 1844.0, 1835.0, 1825.0, 1816.0, 1806.0, 1797.0, 1787.0, 1778.0, 1768.0, 1759.0, 1749.0, 1740.0, 1730.0, 1721.0, 1711.0, 1702.0, 1693.0, 1683.0, 1674.0, 1665.0, 1655.0, 1646.0, 1637.0, 1627.0, 1618.0, 1609.0, 1599.0, 1590.0, 1581.0, 1572.0, 1562.0, 1553.0, 1544.0, 1535.0, 1525.0, 1516.0, 1507.0, 1498.0, 1489.0, 1479.0, 1470.0, 1461.0, 1452.0, 1443.0, 1434.0, 1425.0, 1416.0, 1407.0, 1398.0, 1388.0, 1379.0, 1370.0, 1361.0, 1352.0, 1343.0, 1334.0, 1325.0, 1316.0, 1307.0, 1299.0, 1290.0, 1281.0, 1272.0, 1263.0, 1254.0, 1245.0, 1236.0, 1227.0, 1218.0, 1210.0, 1201.0, 1192.0, 1183.0, 1174.0, 1166.0, 1157.0, 1148.0, 1139.0, 1130.0, 1122.0, 1113.0, 1104.0, 1096.0, 1087.0, 1078.0, 1069.0, 1061.0, 1052.0, 1043.0, 1035.0, 1026.0, 1018.0, 1009.0, 1000.0, 992.0, 983.0, 975.0, 966.0, 958.0, 950.0, 941.0, 933.0, 925.0, 917.0, 908.0, 900.0, 892.0, 884.0, 876.0, 868.0, 860.0, 852.0, 844.0, 837.0, 829.0, 821.0, 813.0, 805.0, 798.0, 790.0, 782.0, 775.0, 767.0, 760.0, 752.0, 745.0, 737.0, 730.0, 722.0, 715.0, 707.0, 700.0, 693.0, 685.0, 678.0, 671.0, 664.0, 656.0, 649.0, 642.0, 635.0, 628.0, 621.0, 613.0, 606.0, 599.0, 592.0, 585.0, 578.0, 571.0, 564.0, 557.0, 550.0, 543.0, 537.0, 530.0, 523.0, 516.0, 509.0, 502.0, 495.0, 489.0, 482.0, 475.0, 468.0, 462.0, 455.0, 448.0, 442.0, 435.0, 428.0, 422.0, 415.0, 408.0, 402.0, 395.0, 389.0, 382.0, 375.0, 369.0, 362.0, 356.0, 349.0, 343.0, 336.0, 330.0, 324.0, 317.0, 311.0, 304.0, 298.0, 291.0, 285.0, 279.0, 272.0, 266.0, 260.0, 253.0, 247.0, 241.0, 234.0, 228.0, 222.0, 215.0, 209.0, 203.0, 197.0, 190.0, 184.0, 178.0, 172.0, 165.0, 159.0, 153.0, 147.0, 141.0, 135.0, 128.0, 122.0, 116.0, 110.0, 104.0, 98.0, 92.0, 85.0, 79.0, 73.0, 67.0, 61.0, 55.0, 49.0, 43.0, 37.0, 31.0, 25.0, 19.0, 13.0, 7.0, 1.0, -5.0, -11.0, -17.0, -23.0, -29.0, -35.0, -41.0, -47.0, -53.0, -59.0, -65.0, -71.0, -77.0, -83.0, -89.0, -95.0, -101.0, -107.0, -113.0, -119.0, -124.0, -130.0, -136.0, -142.0, -148.0, -154.0, -160.0, -166.0, -172.0, -177.0, -183.0, -189.0, -195.0, -201.0, -207.0, -212.0, -218.0, -224.0, -230.0, -236.0, -242.0, -247.0, -253.0, -259.0, -265.0, -271.0, -276.0, -282.0, -288.0, -294.0, -300.0, -305.0, -311.0, -317.0, -323.0, -328.0, -334.0, -340.0, -346.0, -351.0, -357.0, -363.0, -369.0, -374.0, -380.0, -386.0, -392.0, -397.0, -403.0, -409.0, -414.0, -420.0, -426.0, -432.0, -437.0, -443.0, -449.0, -454.0, -460.0, -466.0, -471.0, -477.0, -483.0, -489.0, -494.0, -500.0, -506.0, -511.0, -517.0, -523.0, -528.0, -534.0, -540.0, -545.0, -551.0, -557.0, -562.0, -568.0, -573.0, -579.0, -585.0, -590.0, -596.0, -602.0, -607.0, -613.0, -619.0, -624.0, -630.0, -635.0, -641.0, -647.0, -652.0, -658.0, -664.0, -669.0, -675.0, -680.0, -686.0, -692.0, -697.0, -703.0, -708.0, -714.0, -720.0, -725.0, -731.0, -737.0, -742.0, -748.0, -753.0, -759.0, -764.0, -770.0, -776.0, -781.0, -787.0, -792.0, -798.0, -804.0, -809.0, -815.0, -820.0, -826.0, -831.0, -837.0, -843.0, -848.0, -854.0, -859.0, -865.0, -871.0, -876.0, -882.0, -887.0, -893.0, -898.0, -904.0, -909.0, -915.0, -921.0, -926.0, -932.0, -937.0, -943.0, -948.0, -954.0, -960.0, -965.0, -971.0, -976.0, -982.0, -987.0, -993.0, -998.0, -1004.0, -1009.0, -1015.0, -1021.0, -1026.0, -1032.0, -1037.0, -1043.0, -1048.0, -1054.0, -1059.0, -1065.0, -1070.0, -1076.0, -1082.0, -1087.0, -1093.0, -1098.0, -1104.0, -1109.0, -1115.0, -1120.0, -1126.0, -1131.0, -1137.0, -1142.0, -1148.0, -1154.0, -1159.0, -1165.0, -1170.0, -1176.0, -1181.0, -1187.0, -1192.0, -1198.0, -1203.0, -1209.0, -1214.0, -1220.0, -1225.0, -1231.0, -1237.0, -1242.0, -1248.0, -1253.0, -1259.0, -1264.0, -1270.0, -1275.0, -1281.0, -1286.0, -1292.0, -1297.0, -1303.0, -1308.0, -1314.0, -1319.0, -1325.0, -1331.0, -1336.0, -1342.0, -1347.0, -1353.0, -1358.0, -1364.0, -1369.0, -1375.0, -1380.0, -1386.0, -1391.0, -1397.0, -1402.0, -1408.0, -1413.0, -1419.0, -1424.0, -1430.0, -1435.0, -1441.0, -1447.0, -1452.0, -1458.0, -1463.0, -1469.0, -1474.0, -1480.0, -1485.0, -1491.0, -1496.0, -1502.0, -1507.0, -1513.0, -1518.0, -1524.0, -1529.0, -1535.0, -1540.0, -1546.0, -1551.0, -1557.0, -1563.0, -1568.0, -1574.0, -1579.0, -1585.0, -1590.0, -1596.0, -1601.0, -1607.0, -1612.0, -1618.0, -1623.0, -1629.0, -1634.0, -1640.0, -1645.0, -1651.0, -1656.0, -1662.0, -1667.0, -1673.0, -1678.0, -1684.0, -1689.0, -1695.0, -1701.0, -1706.0, -1712.0, -1717.0, -1723.0, -1728.0, -1734.0, -1739.0, -1745.0, -1750.0, -1756.0, -1761.0, -1767.0, -1772.0, -1778.0, -1783.0, -1789.0, -1794.0, -1800.0, -1805.0, -1811.0, -1816.0, -1822.0, -1827.0, -1833.0, -1838.0, -1844.0, -1849.0, -1855.0, -1861.0, -1866.0, -1872.0, -1877.0, -1883.0, -1888.0, -1894.0, -1899.0, -1905.0, -1910.0, -1916.0, -1921.0, -1927.0, -1932.0, -1938.0, -1943.0, -1949.0, -1954.0, -1960.0, -1965.0, -1971.0, -1976.0, -1982.0, -1987.0, -1993.0, -1998.0, -2004.0, -2009.0, -2015.0, -2020.0, -2026.0, -2031.0, -2037.0, -2042.0, -2048.0, -2047.0, -2035.0, -2024.0, -2012.0, -2001.0, -1989.0, -1977.0, -1966.0, -1954.0, -1943.0, -1931.0, -1920.0, -1908.0, -1897.0, -1886.0, -1874.0, -1863.0, -1851.0, -1840.0, -1829.0, -1817.0, -1806.0, -1795.0, -1783.0, -1772.0, -1761.0, -1750.0, -1738.0, -1727.0, -1716.0, -1705.0, -1694.0, -1683.0, -1671.0, -1660.0, -1649.0, -1638.0, -1627.0, -1616.0, -1605.0, -1594.0, -1583.0, -1572.0, -1561.0, -1550.0, -1539.0, -1528.0, -1517.0, -1507.0, -1496.0, -1485.0, -1474.0, -1463.0, -1452.0, -1442.0, -1431.0, -1420.0, -1409.0, -1399.0, -1388.0, -1377.0, -1367.0, -1356.0, -1345.0, -1335.0, -1324.0, -1314.0, -1303.0, -1293.0, -1282.0, -1271.0, -1261.0, -1250.0, -1240.0, -1230.0, -1219.0, -1209.0, -1198.0, -1188.0, -1178.0, -1167.0, -1157.0, -1147.0, -1136.0, -1126.0, -1116.0, -1105.0, -1095.0, -1085.0, -1075.0, -1065.0, -1054.0, -1044.0, -1034.0, -1024.0, -1014.0, -1004.0, -994.0, -984.0, -974.0, -964.0, -954.0, -944.0, -934.0, -924.0, -914.0, -904.0, -894.0, -884.0, -874.0, -864.0, -854.0, -844.0, -835.0, -825.0, -815.0, -806.0, -796.0, -786.0, -777.0, -768.0, -758.0, -749.0, -740.0, -731.0, -722.0, -713.0, -704.0, -695.0, -686.0, -678.0, -669.0, -660.0, -652.0, -643.0, -635.0, -626.0, -618.0, -610.0, -601.0, -593.0, -585.0, -577.0, -569.0, -561.0, -553.0, -545.0, -537.0, -529.0, -521.0, -513.0, -506.0, -498.0, -490.0, -483.0, -475.0, -467.0, -460.0, -452.0, -445.0, -437.0, -430.0, -423.0, -415.0, -408.0, -401.0, -393.0, -386.0, -379.0, -372.0, -365.0, -358.0, -351.0, -343.0, -336.0, -329.0, -322.0, -316.0, -309.0, -302.0, -295.0, -288.0, -281.0, -274.0, -268.0, -261.0, -254.0, -247.0, -241.0, -234.0, -227.0, -221.0, -214.0, -207.0, -201.0, -194.0, -188.0, -181.0, -175.0, -168.0, -162.0, -155.0, -149.0, -143.0, -136.0, -130.0, -123.0, -117.0, -111.0, -104.0, -98.0, -92.0, -86.0, -79.0, -73.0, -67.0, -61.0, -54.0, -48.0, -42.0, -36.0, -30.0, -24.0, -18.0, -11.0, -5.0, 1.0, 7.0, 13.0, 19.0, 25.0, 31.0, 37.0, 43.0, 49.0, 55.0, 61.0, 67.0, 73.0, 78.0, 84.0, 90.0, 96.0, 102.0, 108.0, 114.0, 120.0, 125.0, 131.0, 137.0, 143.0, 149.0, 154.0, 160.0, 166.0, 172.0, 178.0, 183.0, 189.0, 195.0, 200.0, 206.0, 212.0, 218.0, 223.0, 229.0, 235.0, 240.0, 246.0, 251.0, 257.0, 263.0, 268.0, 274.0, 280.0, 285.0, 291.0, 296.0, 302.0, 307.0, 313.0, 319.0, 324.0, 330.0, 335.0, 341.0, 346.0, 352.0, 357.0, 363.0, 368.0, 374.0, 379.0, 385.0, 390.0, 396.0, 401.0, 407.0, 412.0, 418.0, 423.0, 428.0, 434.0, 439.0, 445.0, 450.0, 455.0, 461.0, 466.0, 472.0, 477.0, 482.0, 488.0, 493.0, 499.0, 504.0, 509.0, 515.0, 520.0, 525.0, 531.0, 536.0, 541.0, 547.0, 552.0, 557.0, 563.0, 568.0, 573.0, 579.0, 584.0, 589.0, 594.0, 600.0, 605.0, 610.0, 616.0, 621.0, 626.0, 631.0, 637.0, 642.0, 647.0, 652.0, 658.0, 663.0, 668.0, 673.0, 678.0, 684.0, 689.0, 694.0, 699.0, 705.0, 710.0, 715.0, 720.0, 725.0, 731.0, 736.0, 741.0, 746.0, 751.0, 757.0, 762.0, 767.0, 772.0, 777.0, 782.0, 788.0, 793.0, 798.0, 803.0, 808.0, 813.0, 818.0, 824.0, 829.0, 834.0, 839.0, 844.0, 849.0, 854.0, 860.0, 865.0, 870.0, 875.0, 880.0, 885.0, 890.0, 895.0, 900.0, 906.0, 911.0, 916.0, 921.0, 926.0, 931.0, 936.0, 941.0, 946.0, 951.0, 956.0, 961.0, 967.0, 972.0, 977.0, 982.0, 987.0, 992.0, 997.0, 1002.0, 1007.0, 1012.0, 1017.0, 1022.0, 1027.0, 1032.0, 1037.0, 1042.0, 1047.0, 1052.0, 1058.0, 1063.0, 1068.0, 1073.0, 1078.0, 1083.0, 1088.0, 1093.0, 1098.0, 1103.0, 1108.0, 1113.0, 1118.0, 1123.0, 1128.0, 1133.0, 1138.0, 1143.0, 1148.0, 1153.0, 1158.0, 1163.0, 1168.0, 1173.0, 1178.0, 1183.0, 1188.0, 1193.0, 1198.0, 1203.0, 1208.0, 1213.0, 1218.0, 1223.0, 1228.0, 1233.0, 1238.0, 1243.0, 1248.0, 1253.0, 1258.0, 1263.0, 1268.0, 1273.0, 1278.0, 1283.0, 1287.0, 1292.0, 1297.0, 1302.0, 1307.0, 1312.0, 1317.0, 1322.0, 1327.0, 1332.0, 1337.0, 1342.0, 1347.0, 1352.0, 1357.0, 1362.0, 1367.0, 1372.0, 1377.0, 1382.0, 1387.0, 1391.0, 1396.0, 1401.0, 1406.0, 1411.0, 1416.0, 1421.0, 1426.0, 1431.0, 1436.0, 1441.0, 1446.0, 1451.0, 1456.0, 1460.0, 1465.0, 1470.0, 1475.0, 1480.0, 1485.0, 1490.0, 1495.0, 1500.0, 1505.0, 1510.0, 1515.0, 1519.0, 1524.0, 1529.0, 1534.0, 1539.0, 1544.0, 1549.0, 1554.0, 1559.0, 1564.0, 1568.0, 1573.0, 1578.0, 1583.0, 1588.0, 1593.0, 1598.0, 1603.0, 1608.0, 1612.0, 1617.0, 1622.0, 1627.0, 1632.0, 1637.0, 1642.0, 1647.0, 1652.0, 1656.0, 1661.0, 1666.0, 1671.0, 1676.0, 1681.0, 1686.0, 1691.0, 1695.0, 1700.0, 1705.0, 1710.0, 1715.0, 1720.0, 1725.0, 1729.0, 1734.0, 1739.0, 1744.0, 1749.0, 1754.0, 1759.0, 1763.0, 1768.0, 1773.0, 1778.0, 1783.0, 1788.0, 1793.0, 1797.0, 1802.0, 1807.0, 1812.0, 1817.0, 1822.0, 1826.0, 1831.0, 1836.0, 1841.0, 1846.0, 1851.0, 1856.0, 1860.0, 1865.0, 1870.0, 1875.0, 1880.0, 1884.0, 1889.0, 1894.0, 1899.0, 1904.0, 1909.0, 1913.0, 1918.0, 1923.0, 1928.0, 1933.0, 1938.0, 1942.0, 1947.0, 1952.0, 1957.0, 1962.0, 1966.0, 1971.0, 1976.0, 1981.0, 1986.0, 1990.0, 1995.0, 2000.0, 2005.0, 2010.0, 2014.0, 2019.0, 2024.0, 2029.0, 2034.0, 2038.0, 2043.0, 2048.0] ("Complete SkewTri")
      # "no smooth"
      # "smooth"
      # "24-09"
      n3 = xnode "Open FPGA VI Reference"() -> ("FPGA VI Reference Out"=w65:refnum<k20>, "error out"=w66:errorcluster)  [unwired: 2 in]
    }
  }
  n4 = Add(x="lower limit 1", y=w56) -> (x+y=w58:u32)
  n5 = Add(x="lower limit 2", y=w56) -> (x+y=w57:u32)
  n6 = xnode "Read/Write Control"("FPGA VI Reference In"=w55, "error in"=w54, "upper limit 1"=w58, "upper limit 2"=w57, "lower limit 1"="lower limit 1", "lower limit 2"="lower limit 2", "Latency points"="Initial Latency points") -> ("FPGA VI Reference Out"=w51:refnum<k20>, "error out"=w50:errorcluster)
  n7 = xnode "Invoke Method"("FPGA VI Reference In"=w51, "error in"=w50, "Requested Depth"=u32 2000) -> ("FPGA VI Reference Out"=w29:refnum<k20>, "error out"=w30:errorcluster)  [unwired: 1 out]
  n8 = xnode "Invoke Method"("FPGA VI Reference In"=w29, "error in"=w30, "Requested Depth"=u32 5000) -> ("FPGA VI Reference Out"=w43:refnum<k20>, "error out"=w44:errorcluster)  [unwired: 1 out]
  n9 = xnode "Invoke Method"("FPGA VI Reference In"=w43, "error in"=w44) -> ("FPGA VI Reference Out"=w27:refnum<k20>, "error out"=w28:errorcluster)
  n10 = xnode "Invoke Method"("FPGA VI Reference In"=w27, "error in"=w28) -> ("FPGA VI Reference Out"=w41:refnum<k20>, "error out"=w42:errorcluster)
  n11 = xnode "Invoke Method"("FPGA VI Reference In"=w41, "error in"=w42) -> ("FPGA VI Reference Out"=w47:refnum<k20>, "error out"=w46:errorcluster)  [unwired: 1 in]
  n12 = Multiply(x=w1, y="Scaling Factor") -> (x*y=w5:dbl[])
  n13 = Array Max & Min(array=w5) -> (max value=w7:dbl)  [unwired: 3 out]
  n14 = Subtract(x=2047.0 ("y"), y=w7) -> (x-y=w6:dbl)
  n15 = Add(x=w6, y=w5) -> (x+y=w4:dbl[])
  n16 = call "Wave Memory write from DMA - Host.vi"("Custom Triangular Signal (fal-ris)"=w4, "Triangolo dritto?"="Triangolo dritto", "error in"=w46, "FPGA VI Reference In"=w47) -> ("FPGA VI Reference Out"=w32:refnum<k20>, "error out"=w45:errorcluster)  [unwired: 5 in, 1 out]
  n17 = call "Window Memory write from DMA - Host.vi"("error in"=w45, "Enum"="Windowing", "FPGA VI Reference In"=w32) -> ("FPGA VI Reference Out"=w53:refnum<k20>, "error out"=w52:errorcluster)  [unwired: 5 in, 2 out]
  n18 = Subtract(x="lower limit 2", y=u32 625) -> (x-y=w13:u32)
  n19 = RT FIFO Create(1:dbl[] [] ("double precision float"), 4:u32 2000 ("size (10)"), 6:u32 1024 ("elements in array (1)")) -> (8:w19:refnum<k33>, 11:w21:errorcluster)  [unwired: 5 in, 1 out]
  n20 = node-c288(i64 2 ("Period")) -> (w40:T2)  [unwired: 3 in]
  n21 = while {
    shift-right: [w70] -> w18
    shift-left: w21 -> [w72]
    tunnel: w19 -> [w77]
    shift-right: [w71] -> _
    shift-left: 0 -> [w75]
    tunnel: "lower limit 1" -> [w67]
    tunnel: w13 -> [w68]
    tunnel: w2 -> [w69]
    stop <- w76 stop-if-true
    # "Non Deterministic Loop (Linearization)"
    n22 = RT FIFO Read(0:w77, 3:w72) -> (9:w74:dbl[], 10:w73:bool, 11:w70:errorcluster)  [unwired: 2 in, 2 out]
    n23 = Wait (ms)(milliseconds to wait=u32 10 ("millisecond multiple")) -> ()  [unwired: 1 out]
    n24 = case shown="False" w73 {
      tunnel: w75 -> [w107 w170]
      tunnel: [w96 w170] -> w71
      tunnel: w74 -> [w105 _]
      tunnel: w69 -> [w86 _]
      tunnel: w68 -> [w83 _]
      tunnel: w67 -> [w82 _]
      frame False {
        n25 = Split 1D Array(array=w105, index=512) -> (first subarray=w94:dbl[], second subarray=w93:dbl[])
        n26 = case shown="True" "Acrive Fit" {
          tunnel: w94 -> [w109 w123]
          tunnel: w93 -> [w108 w119]
          tunnel: "Poly Grade" -> [_ w115]
          tunnel: "Side points" -> [_ w114]
          tunnel: "Poly Order" -> [_ w113]
          tunnel: [w108 w112] -> w87
          tunnel: [w109 w110] -> w88
          tunnel: "Acrive  Smooth" -> [_ w111]
          frame False {
          }
          frame True {
            n27 = call "Poly Fitting.vi"("Poly Grade"=w115, "Signal"=w123) -> ("Poly Signal"=w122:dbl[], "SubtractedSignal"=w117:dbl[])  [unwired: 8 in]
            n28 = call "Poly Fitting.vi"("Poly Grade"=w115, "Signal"=w119) -> ("Poly Signal"=w118:dbl[], "SubtractedSignal"=w116:dbl[])  [unwired: 8 in]
            n29 = Build Array(w123, w122) -> (→"1) Signal&Fit":dbl[][])
            n30 = Build Array(w119, w118) -> (→"2) Signal&Fit 2":dbl[][])
            n31 = case shown="True" w111 {
              tunnel: w117 -> [w125 w131]
              tunnel: w116 -> [w124 w130]
              tunnel: w114 -> [_ w129]
              tunnel: w113 -> [_ w128]
              tunnel: [w124 w127] -> w112
              tunnel: [w125 w126] -> w110
              frame False {
              }
              frame True {
                n32 = call "Smoothing.vi"("polynomial order"=w128, "side points"=w129, "SubtractedSignal"=w131) -> ("SubSmoothSignal"=w126:dbl[])  [unwired: 8 in]
                "1) SmoothSubSig" <- w126
                n33 = call "Smoothing.vi"("polynomial order"=w128, "side points"=w129, "SubtractedSignal"=w130) -> ("SubSmoothSignal"=w127:dbl[])  [unwired: 8 in]
                "2) SmoothSubSig" <- w127
              }
            }
          }
        }
        n34 = call "Sliding FFT.vi"("Sample Freq"=w86, "FFT Win Size"="FFT Sliding Win Size", "SubSmoothSignal"=w88) -> ("Freq samples"=w85:dbl[])  [unwired: 7 in, 1 out]
        "1) Freq curve" <- w85
        n35 = call "Sliding FFT.vi"("Sample Freq"=w86, "FFT Win Size"="FFT Sliding Win Size", "SubSmoothSignal"=w87) -> ("Freq samples"=w84:dbl[])  [unwired: 7 in, 1 out]
        "2) Freq curve" <- w84
        n36 = Increment(x=w107) -> (x+1=w97:i32)
        "Current Sig lin" <- w97
        n37 = Equal?(x=1, y=w97) -> (x = y?=w103:bool)
        n38 = feedback #1() -> (w102:T5)  [unwired: 1 in]
        n39 = feedback #2() -> (w101:T5)  [unwired: 1 in]
        n40 = case shown="False" w103 {
          tunnel: w84 -> [w164 w167]
          tunnel: w85 -> [w165 w169]
          tunnel: [w163 w166] -> w98
          tunnel: [w162 w168] -> w99
          tunnel: w102 -> [w161 _]
          tunnel: w101 -> [w160 _]
          frame False {
            n41 = Build Array (concatenate)(w161, w165) -> (w162:T5)
            n42 = Build Array (concatenate)(w160, w164) -> (w163:T5)
          }
          frame True {
            n43 = Build Array(w169) -> (w168:T5)
            n44 = Build Array(w167) -> (w166:T5)
          }
        }
        n45 = feedback-in #1(w99) -> ()
        n46 = feedback-in #2(w98) -> ()
        n47 = Equal?(x="# Measurements for Linearization", y=w97) -> (x = y?=w95:bool)
        n48 = case shown="True" w95 {
          tunnel: w99 -> [_ w142]
          tunnel: w98 -> [_ w141]
          tunnel: w97 -> [w132 _]
          tunnel: [w132 0] -> w96
          tunnel: w83 -> [_ w154]
          tunnel: w82 -> [_ w153]
          tunnel: "FFT Sliding Win Size" -> [_ w152]
          tunnel: "Active PolyFit" -> [_ w134]
          tunnel: "Active PolyFit" -> [_ w133]
          frame False {
          }
          frame True {
            n49 = call "Mean Freq Curves.vi"("Set of Freq samples"=w141, "Active Fit"=w133) -> ("Mean Freq Curve"=w140:dbl[], "Max-Min error (% over Mean)"=→"2) Max-Min error":dbl, "StdDev%"=→"2) Std Dev":dbl)  [unwired: 12 in, 3 out]
            "2) Mean Freq Curve Rising" <- w140
            n50 = call "Mean Freq Curves.vi"("Set of Freq samples"=w142, "Active Fit"=w134) -> ("Mean Freq Curve"=w138:dbl[], "Max-Min error (% over Mean)"=→"1) Max-Min error":dbl, "StdDev%"=→"1) Std Dev":dbl)  [unwired: 12 in, 3 out]
            "1) Mean Freq Curve Falling" <- w138
            n51 = Reciprocal(x=w140) -> (1/x=w149:dbl[])
            n52 = Reciprocal(x=w138) -> (1/x=w148:dbl[])
            n53 = call "AdjusteExtremeCurve.vi"("Init Bins Discarded"=w154, "FFT Size Window"=w152, "Freq sample"=w149) -> ("Extended Freq Sample"=w150:dbl[])  [unwired: 8 in]
            "2) Ext Mean Time Curve" <- w150
            n54 = call "AdjusteExtremeCurve.vi"("Init Bins Discarded"=w153, "FFT Size Window"=w152, "Freq sample"=w148) -> ("Extended Freq Sample"=w151:dbl[])  [unwired: 8 in]
            "1) Ext Mean Time Curve" <- w151
            n55 = call "Triangular Egde Generator.vi"("fattore"="Scale Factor Falling", "Sample values"=w151, "Triangular edge"=enum16{"Rising", "Falling"}."Falling") -> ("Skew Triangular"=w156:dbl[])  [unwired: 8 in]
            "1) Tri edge FALLING" <- w156
            n56 = call "Triangular Egde Generator.vi"("fattore"="Scale Factor Rising", "Sample values"=w150, "Triangular edge"=enum16{"Rising", "Falling"}."Falling") -> ("Skew Triangular"=w146:dbl[])  [unwired: 8 in]
            n57 = Multiply(x=w146, y=-1.0) -> (x*y=w145:dbl[])
            "2) Tri edge RISING" <- w145
            n58 = Build Array (concatenate)(w156, w145) -> (→"Complete SkewTri":dbl[])
          }
        }
      }
      frame True {
      }
    }
    n59 = local read item#18() -> (w76:bool)
  }
  n60 = timed-loop {
    tunnel: w53 -> [w197]
    tunnel: w52 -> [w198]
    tunnel: [w200] -> w37
    tunnel: w2 -> [w202]
    tunnel: [w201] -> w36
    timing: w40 -> [_]
    timing-out: [_] -> w39
    tunnel: "first bin" -> [w186]
    tunnel: "last bin" -> [w185]
    tunnel: [w183] -> w31
    tunnel: "Windowing" -> [w181]
    shift-right: [w175] -> w22
    shift-left: w21 -> [w177]
    tunnel: w19 -> [w179]
    shift-right: [w171] -> _
    shift-left: 0 -> [w173]
    stop <- "?" stop-if-true
    # "Deterministic Loop (Signal and FFT Read)"
    n61 = node-c288() -> ()  [unwired: 1 in, 1 out]
    n62 = flat-sequence {
      tunnel: w197 -> [w210]
      tunnel: w198 -> [w211]
      tunnel: "Snapshot" -> [w208]
      tunnel: "Snapshot" -> [w213]
      tunnel: w202 -> [w214]
      tunnel: [w212] -> w196
      tunnel: [w214] -> w195
      tunnel: [w213] -> w194
      tunnel: [w208] -> w193
      tunnel: [w212] -> w192
      tunnel: [w209] -> w191
      tunnel: [w209] -> w190
      tunnel: [w207] -> w180
      tunnel: w179 -> [w207]
      tunnel: [w206] -> w178
      tunnel: w177 -> [w206]
      tunnel: [w205] -> w174
      tunnel: w173 -> [w205]
      tunnel: w196 -> [w239]
      tunnel: w195 -> [w227]
      tunnel: w194 -> [w233]
      tunnel: w193 -> [w236]
      tunnel: w192 -> [w235]
      tunnel: w191 -> [w234]
      tunnel: w190 -> [w240]
      tunnel: [w238] -> w189
      tunnel: [w237] -> w188
      tunnel: [w232] -> w187
      tunnel: w186 -> [w231]
      tunnel: w185 -> [w230]
      tunnel: [w229] -> w182
      tunnel: w181 -> [w228]
      tunnel: w180 -> [w226]
      tunnel: w178 -> [w225]
      tunnel: [w223] -> w176
      tunnel: w174 -> [w222]
      tunnel: [w222] -> w172
      tunnel: [w335] -> w200
      tunnel: [w336] -> w201
      tunnel: w189 -> [w336]
      tunnel: w188 -> [w335]
      tunnel: w187 -> [w334]
      tunnel: [w333] -> w183
      tunnel: w182 -> [w333]
      tunnel: [w332] -> w175
      tunnel: w176 -> [w332]
      tunnel: w172 -> [w331]
      tunnel: [w330] -> w171
      frame #0 {
        n63 = case shown="True" w208 {
          tunnel: [w215 w220] -> w212
          tunnel: w211 -> [w215 w219]
          tunnel: w210 -> [w216 w218]
          tunnel: [w216 w217] -> w209
          frame False {
          }
          frame True {
            n64 = xnode "Read/Write Control"("FPGA VI Reference In"=w218, "error in"=w219, "snapshot"=TRUE) -> ("FPGA VI Reference Out"=w217:refnum<k20>, "error out"=w220:errorcluster)
          }
        }
      }
      frame #1 {
        n65 = flat-sequence {
          tunnel: w240 -> [w252]
          tunnel: w239 -> [w251]
          tunnel: w227 -> [w250]
          tunnel: w233 -> [w247]
          tunnel: [w249] -> w243
          tunnel: [w248] -> w242
          tunnel: [w247] -> w241
          tunnel: w226 -> [w246]
          tunnel: w225 -> [w245]
          tunnel: [w244] -> w224
          tunnel: [w288] -> w237
          tunnel: w243 -> [w290]
          tunnel: w242 -> [w289]
          tunnel: w241 -> [w287]
          tunnel: [w287] -> w232
          tunnel: [w286] -> w229
          tunnel: [w285] -> w223
          tunnel: w224 -> [w285]
          frame #0 {
            n66 = case shown="True" w247 {
              tunnel: w252 -> [w260 w279]
              tunnel: w251 -> [w258 w278]
              tunnel: [w257 w271] -> w248
              tunnel: w250 -> [_ _]
              tunnel: [w254 w270] -> w249
              tunnel: w246 -> [_ w265]
              tunnel: w245 -> [w253 w264]
              tunnel: [w253 w263] -> w244
              frame False {
                n67 = xnode "Invoke Method"("FPGA VI Reference In"=w260, "error in"=w258, "Number of Elements"=u32 0) -> ("FPGA VI Reference Out"=w256:refnum<k20>, "error out"=w255:errorcluster, "Elements Remaining"=w259:u32)  [unwired: 1 in, 1 out]
                n68 = xnode "Invoke Method"("FPGA VI Reference In"=w256, "error in"=w255, "Number of Elements"=w259) -> ("FPGA VI Reference Out"=w254:refnum<k20>, "error out"=w257:errorcluster)  [unwired: 1 in, 2 out]
              }
              frame True {
                n69 = xnode "Invoke Method"("FPGA VI Reference In"=w279, "error in"=w278, "Number of Elements"=u32 1024, "Timeout (ms)"=-1) -> ("FPGA VI Reference Out"=w273:refnum<k20>, "error out"=w272:errorcluster, "Data"=w275:fxp<+/-,12,12>[])  [unwired: 1 out]
                n70 = To Double Precision Float(number=w275) -> (double precision float=w266:dbl[])
                n71 = case shown="True" "Acrive Linearization" {
                  tunnel: w266 -> [_ w284]
                  tunnel: w265 -> [_ w283]
                  tunnel: w264 -> [w280 w282]
                  tunnel: [w280 w281] -> w263
                  frame False {
                  }
                  frame True {
                    n72 = RT FIFO Write(0:w283, 1:w284, 3:w282) -> (11:w281:errorcluster)  [unwired: 2 in, 3 out]
                  }
                }
                n73 = Split 1D Array(array=w266, index=512) -> (first subarray=→"First Signal (points) - Falling Triangular":dbl[], second subarray=→"Second Signal (points) - Rising Triangular":dbl[])
                n74 = xnode "Invoke Method"("FPGA VI Reference In"=w273, "error in"=w272, "Number of Elements"=u32 0) -> ("FPGA VI Reference Out"=w270:refnum<k20>, "error out"=w271:errorcluster)  [unwired: 1 in, 2 out]
              }
            }
          }
          frame #1 {
            n75 = case shown="True" w287 {
              tunnel: [w292 w295] -> w288
              tunnel: w290 -> [w291 w296]
              tunnel: w289 -> [w292 w294]
              tunnel: [w291 w293] -> w286
              frame False {
              }
              frame True {
                n76 = xnode "Read/Write Control"("FPGA VI Reference In"=w296, "error in"=w294, "snapshot"=FALSE) -> ("FPGA VI Reference Out"=w293:refnum<k20>, "error out"=w295:errorcluster)
              }
            }
          }
        }
        n77 = case shown="True" w236 {
          tunnel: w234 -> [w303 w324]
          tunnel: w235 -> [w300 w325]
          tunnel: [w299 w323] -> w238
          tunnel: w231 -> [_ w310]
          tunnel: w230 -> [_ w311]
          tunnel: w228 -> [_ w307]
          tunnel: w227 -> [_ w305]
          frame False {
            n78 = xnode "Invoke Method"("FPGA VI Reference In"=w303, "error in"=w300, "Number of Elements"=u32 0) -> ("FPGA VI Reference Out"=w301:refnum<k20>, "error out"=w298:errorcluster, "Elements Remaining"=w302:u32)  [unwired: 1 in, 1 out]
            n79 = xnode "Invoke Method"("FPGA VI Reference In"=w301, "error in"=w298, "Number of Elements"=w302) -> ("error out"=w299:errorcluster)  [unwired: 1 in, 3 out]
          }
          frame True {
            n80 = xnode "Invoke Method"("FPGA VI Reference In"=w324, "error in"=w325, "Number of Elements"=u32 512, "Timeout (ms)"=-1) -> ("FPGA VI Reference Out"=w321:refnum<k20>, "error out"=w322:errorcluster, "Data"=w327:fxp<+,44,44>[])  [unwired: 1 out]
            n81 = To Double Precision Float(number=w327) -> (double precision float=w326:dbl[])
            n82 = Square Root(x=w326) -> (sqrt(x)=w319:dbl[])
            n83 = Split 1D Array(array=w319, index=256) -> (first subarray=w317:dbl[], second subarray=w316:dbl[])
            "First FFT (bin)" <- w317
            "Second FFT (bin)" <- w316
            n84 = xnode "Invoke Method"("FPGA VI Reference In"=w321, "error in"=w322, "Number of Elements"=u32 0) -> ("error out"=w323:errorcluster)  [unwired: 1 in, 3 out]
            n85 = call "Distance-Velocity Calculation RT.vi"("First FFT"=w317, "Second FFT"=w316, "Windowing"=w307, "first FFT bin"=w310, "Sample Rate (S/s)"=w305, "last FFT bin"=w311) -> ("F_rise"=→"f_rise":dbl, "maxbin_firstFFT"=→"maxbin_firstFFT":i32, "maxbin_secondFFT"=→"maxbin_secondFFT":i32, "Distance (m)"=→"Distance (m)":dbl, "f_mean"=→"f_mean":dbl, "F_fall"=→"f_fall":dbl, "Velocity (m/s)"=→"Velocity (m/s)":dbl)  [unwired: 7 in]
          }
        }
      }
      frame #2 {
        n86 = case shown="True" w334 {
          tunnel: w331 -> [w337 w341]
          tunnel: [w337 w342] -> w330
          frame False {
          }
          frame True {
            n87 = Decrement(x="tieni premuto per") -> (x-1=w338:i32)
            n88 = Greater Or Equal?(x=w341, y=w338) -> (x >= y?=w340:bool)
            n89 = case shown="True" w340 {
              tunnel: w341 -> [w343 _]
              tunnel: [w344 0] -> w342
              frame False {
                n90 = Increment(x=w343) -> (x+1=w344:i32)
              }
              frame True {
                n91 = local write "Snapshot"(FALSE ("Snapshot")) -> ()
              }
            }
          }
        }
      }
    }
    n92 = node-c288() -> ()  [unwired: 1 in, 1 out]
  }
  n93 = node-c288(w39) -> ()  [unwired: 1 out]
  n94 = RT FIFO Delete(0:w19, 3:w18) -> (11:w17:errorcluster)  [unwired: 1 in]
  n95 = Merge Errors(w36, w37, w22, w17) -> (w20:errorcluster)
  n96 = flat-sequence {
    tunnel: w20 -> [w350]
    tunnel: w31 -> [w347]
    frame #0 {
      n97 = property class="Bool (strict)"(error in=w350, "Value"=FALSE ("stop")) -> (error out=w349:errorcluster)  [unwired: 1 in, 1 out]
      n98 = xnode "Invoke Method"("FPGA VI Reference In"=w347, "error in"=w349) -> ("FPGA VI Reference Out"=w352:refnum<k20>, "error out"=w351:errorcluster)
      n99 = xnode "Invoke Method"("FPGA VI Reference In"=w352, "error in"=w351) -> ("FPGA VI Reference Out"=w353:refnum<k20>, "error out"=w354:errorcluster)
      n100 = xnode "Close FPGA VI Reference"("FPGA VI Reference In"=w353, "error in"=w354) -> ()  [unwired: 1 out]
    }
  }
